vi "Is Dynamic Dispatch.vi"(8 "error in (no error)":errorcluster, 11 "Data in":T1) -> (0 "error out":errorcluster, 2 "Is Dynamic Dispatch?":bool, 3 "Data out":T1)   [LabVIEW 2020, in "Peek Window.lvlib" / "Dynamic Dispatch VI Type.lvclass"]
uses:
  Dynamic Dispatch VI Type.lvclass
  MHL Data Cluster.ctl
  Standard VI Type/Standard VI Type.lvclass
  Standard VI Type/Standard VI Type.lvclass/Standard VI Type.ctl
  Standard VI Type/Read VI Refnum.vi
  Dynamic Dispatch VI Type.lvclass/Dynamic Dispatch VI Type.ctl
  Peek Window.lvlib
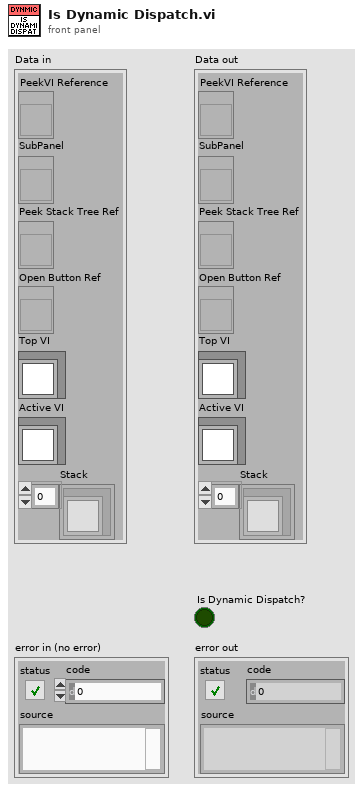
[diagram p1: front panel]
types:
  T1 = typedef "Peek Window.lvlib/MHL Data Cluster.ctl" = cluster{"PeekVI Reference":refnum<vi>, "SubPanel":refnum<vi>, "Peek Stack Tree Ref":refnum<vi>, "Open Button Ref":refnum<vi>, "Top VI":refnum<class "Standard VI Type.lvclass">, "Active VI":refnum<class "Standard VI Type.lvclass">, "Stack":refnum<class "Standard VI Type.lvclass">[]}
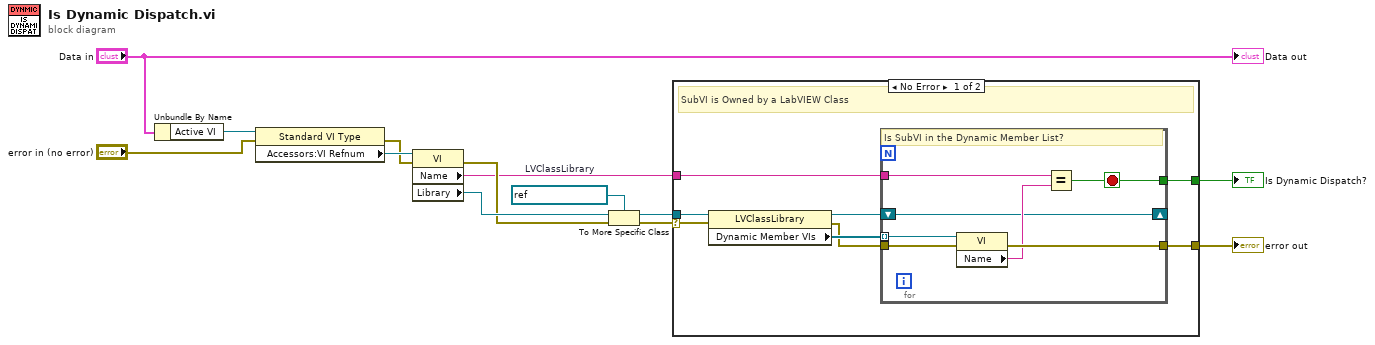
[diagram p0: block diagram]
diagram:
  w13 = refnum<vi> refnum  # LVClassLibrary
  n1 = Unbundle By Name("Data in") -> ("Active VI"=w4:refnum<class "Standard VI Type.lvclass">)
  n2 = property class="Standard VI Type"(reference=w4, error in="error in (no error)") -> (error out=w1:errorcluster, "Accessors:VI Refnum"=w3:refnum<vi>)  [unwired: 1 out]
  n3 = property class="VI"(reference=w3, error in=w1) -> (error out=w8:errorcluster, "Name"=w6:string, "Library"=w9:refnum<vi>)  [unwired: 1 out]
  n4 = To More Specific Class(target class=w13, reference=w9, error in=w8) -> (specific class reference=w12:refnum<vi>, error out=w11:errorcluster)
  n5 = case shown="No Error" w11 {
    selector: w11 -> [w20 _]
    tunnel: w12 -> [w21 _]
    tunnel: w6 -> [w19 _]
    tunnel: [w15 _] -> w10
    tunnel: [w14 _] -> w5
    frame No Error {
      # "SubVI is Owned by a LabVIEW Class"
      n6 = property class="LVClassLibrary"(reference=w21, error in=w20) -> (reference out=w16:refnum<vi>, error out=w17:errorcluster, "Dynamic Member VIs"=w18:refnum<vi>[])
      n7 = for {
        tunnel: w19 -> [w27]
        tunnel: w18 -> [w28] mode=indexing
        tunnel: w17 -> [w26]
        tunnel: [w25] -> w14
        tunnel: [w24] -> w15
        shift-right: [w22] -> _
        shift-left: w16 -> [w22]
        stop <- w24 stop-if-true
        # "Is SubVI in the Dynamic Member List?"
        n8 = property class="VI"(reference=w28, error in=w26) -> (error out=w25:errorcluster, "Name"=w23:string)  [unwired: 1 out]
        n9 = Equal?(x=w27, y=w23) -> (x = y?=w24:bool)
      }
    }
    frame Error {
      # "Not in a Class or in a Library"
    }
  }
  "error out" <- w5
  "Is Dynamic Dispatch?" <- w10
  "Data out" <- "Data in"
